vi "set_As_gas.vi"(0 "Active":bool, 1 "As_Gas Flow":dbl, 5 "Gas In":bool, 7 "H2 Flush":bool, 9 "Run":bool, 11 "Remote":bool=TRUE) -> ()   [LabVIEW 2011]
uses:
  low_level_proc/globals.vi
  editor_lib/Flow_Globals.vi
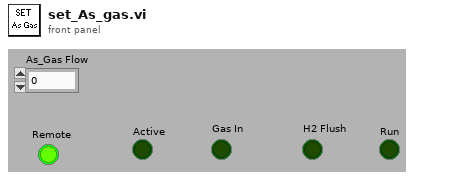
[diagram p1: front panel]
types:
  T1 = typedef "relaySpec.ctl" = cluster{"Card Index":u16, "Relay Index":u16}
  T2 = typedef "DA_Spec.ctl" = cluster{"Card Index":u16, "Channel Index":u16}
  T3 = typedef "AD_Spec.ctl" = u16
  T4 = cluster{"Relay Functions":cluster{"Remote":T1, "Active":T1, "Gas in":T1, "H2 flush":T1, "Run":T1}, "D/A Functions":cluster{"Flow":T2}, "Flow Range":cluster{"Flow (ASGMFC1)":u16}, "A/D Functions":cluster{"Flow":T3}}
  T5 = cluster{"Remote":T1, "Active":T1, "Gas in":T1, "H2 flush":T1, "Run":T1}
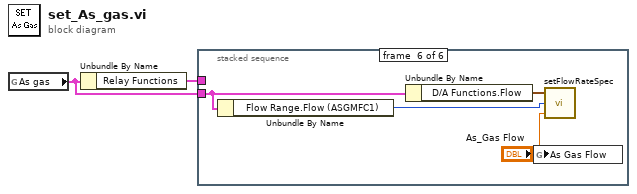
[diagram p0: block diagram]
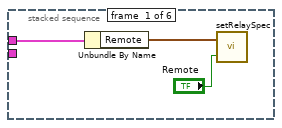
[diagram p2: hidden frame]
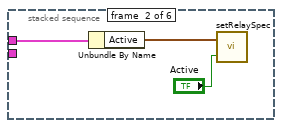
[diagram p3: hidden frame]
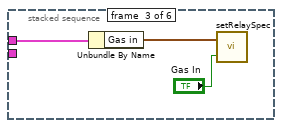
[diagram p4: hidden frame]
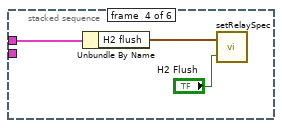
[diagram p5: hidden frame]
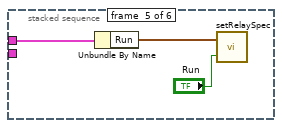
[diagram p6: hidden frame]
diagram:
  n1 = global read "globals.vi" "As gas"() -> (w1:T4)
  n2 = Unbundle By Name(w1) -> ("Relay Functions"=w2:T5)
  n3 = stacked-sequence {
    tunnel: w2 -> [w3 w7 w9 w13 w16 _]
    tunnel: w1 -> [_ _ _ _ _ w21]
    frame #0 {
      n4 = Unbundle By Name(w3) -> ("Remote"=w5:T1)
      n5 = call "setRelaySpec.vi"("Relay Status"="Remote", "RelaySpec"=w5) -> ()  [unwired: 1 in]
    }
    frame #1 {
      n6 = Unbundle By Name(w7) -> ("Active"=w8:T1)
      n7 = call "setRelaySpec.vi"("Relay Status"="Active", "RelaySpec"=w8) -> ()  [unwired: 1 in]
    }
    frame #2 {
      n8 = Unbundle By Name(w9) -> ("Gas in"=w11:T1)
      n9 = call "setRelaySpec.vi"("Relay Status"="Gas In", "RelaySpec"=w11) -> ()  [unwired: 1 in]
    }
    frame #3 {
      n10 = Unbundle By Name(w13) -> ("H2 flush"=w14:T1)
      n11 = call "setRelaySpec.vi"("Relay Status"="H2 Flush", "RelaySpec"=w14) -> ()  [unwired: 1 in]
    }
    frame #4 {
      n12 = Unbundle By Name(w16) -> ("Run"=w15:T1)
      n13 = call "setRelaySpec.vi"("Relay Status"="Run", "RelaySpec"=w15) -> ()  [unwired: 1 in]
    }
    frame #5 {
      n14 = Unbundle By Name(w21) -> ("Flow Range.Flow (ASGMFC1)"=w19:u16)
      n15 = Unbundle By Name(w21) -> ("D/A Functions.Flow"=w20:T2)
      n16 = global write "Flow_Globals.vi" "As Gas Flow"("As_Gas Flow") -> ()
      n17 = call "setFlowRateSpec.vi"("Flow Rate (sccm)"="As_Gas Flow", "Flow range Index"=w19, "D/A Card"=w20) -> ()  [unwired: 2 in]
    }
  }
